vi "Insert Into Subpanel.vi"(8 "error in (no error)":errorcluster, 10 "Key":string, 11 "Subpanel.lvclass":refnum<class "Subpanel.lvclass">) -> (0 "error out":errorcluster, 3 "Subpanel out":refnum<class "Subpanel.lvclass">)   [LabVIEW 2019, in "Subpanel.lvclass"]
uses:
  Subpanel.lvclass
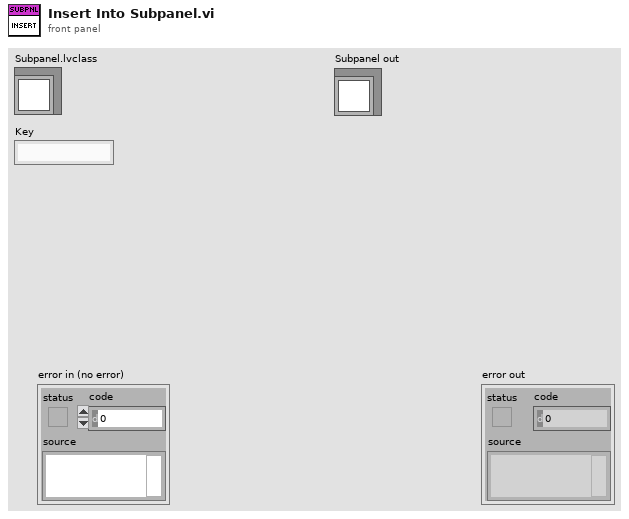
[diagram p1: front panel]
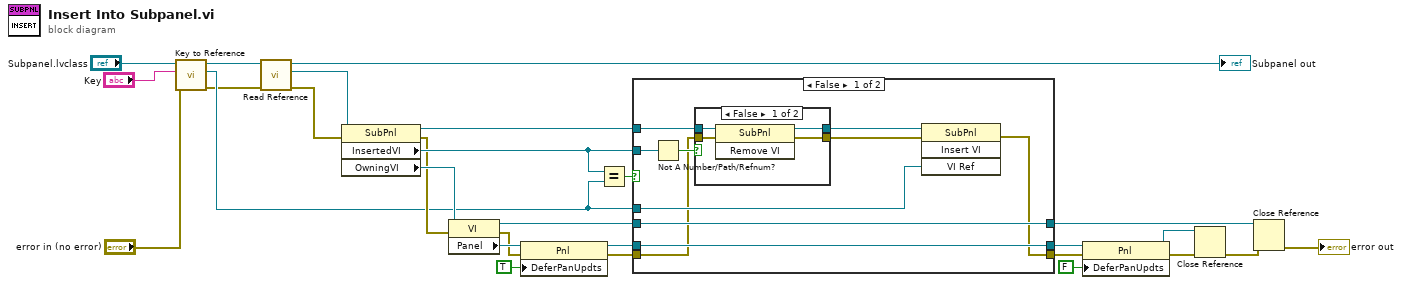
[diagram p0: block diagram]
diagram:
  n1 = call-dynamic "Key to Reference.vi"("error in (no error)"="error in (no error)", "Key"="Key", "Subpanel in"="Subpanel.lvclass") -> ("error out"=w2:errorcluster, "Reference"=w7:refnum<vi>, "Subpanel out"=w4:refnum<class "Subpanel.lvclass">)  [unwired: 6 in]
  n2 = call-dynamic "Read Reference.vi"("error in (no error)"=w2, "Subpanel in"=w4) -> ("error out"=w1:errorcluster, "Reference"=w5:refnum<vi>, "Subpanel out"=→"Subpanel out":refnum<class "Subpanel.lvclass">)  [unwired: 7 in]
  n3 = property class="SubPnl"(reference=w5, error in=w1) -> (reference out=w27:refnum<vi>, error out=w11:errorcluster, "InsertedVI"=w26:refnum<vi>, "OwningVI"=w21:refnum<vi>)
  n4 = property class="VI"(reference=w21, error in=w11) -> (reference out=w22:refnum<vi>, error out=w24:errorcluster, "Panel"=w25:refnum<vi>)
  n5 = property class="Pnl"(reference=w25, error in=w24, "DeferPanUpdts"=TRUE ("Defer Panel Updates")) -> (reference out=w23:refnum<vi>, error out=w10:errorcluster)
  n6 = Equal?(x=w26, y=w7) -> (x = y?=w28:bool)
  n7 = case shown="False" w28 {
    tunnel: w27 -> [w38 _]
    tunnel: w7 -> [w34 _]
    tunnel: w26 -> [w37 _]
    tunnel: w10 -> [w31 w45]
    tunnel: [w33 w46] -> w20
    tunnel: w23 -> [w33 w46]
    tunnel: [w32 w47] -> w17
    tunnel: w22 -> [w32 w47]
    tunnel: [w30 w45] -> w12
    frame False {
      n8 = Not A Number/Path/Refnum?(number/path/refnum=w37) -> (NaN/Path/Refnum?=w36:bool)
      n9 = case shown="False" w36 {
        tunnel: w38 -> [w42 w44]
        tunnel: [w41 w44] -> w35
        tunnel: [w40 w43] -> w29
        tunnel: w31 -> [w39 w43]
        frame False {
          n10 = invoke class="SubPnl" method="Remove VI"(reference=w42, error in=w39) -> (reference out=w41:refnum<vi>, error out=w40:errorcluster)  [unwired: 1 in, 1 out]
        }
        frame True {
        }
      }
      n11 = invoke class="SubPnl" method="Insert VI"(reference=w35, error in=w29, "VI Ref"=w34) -> (error out=w30:errorcluster)  [unwired: 1 in, 3 out]
    }
    frame True {
    }
  }
  n12 = property class="Pnl"(reference=w20, error in=w12, "DeferPanUpdts"=FALSE ("Defer Panel Updates")) -> (reference out=w19:refnum<vi>, error out=w18:errorcluster)
  n13 = Close Reference(reference=w19, error in (no error)=w18) -> (error out=w16:errorcluster)
  n14 = Close Reference(reference=w17, error in (no error)=w16) -> (error out=→"error out":errorcluster)
